vi "Write appended array.vi"(8 "error in (no error)":errorcluster, 10 "appended array":cluster{"AI Channel Data":T1[]}[](array[cluster]), 11 "DAQ Data in":refnum<class "DAQ Data.lvclass">) -> (0 "error out":errorcluster, 3 "DAQ Data out":refnum<class "DAQ Data.lvclass">)   [LabVIEW 2022 SP3, in "DAQ Data.lvclass"]
uses:
  DAQ Data.lvclass
  AIDAQ Data.ctl
  DAQ Data.lvclass/DAQ Data.ctl
  AI Daq Data.lvlib
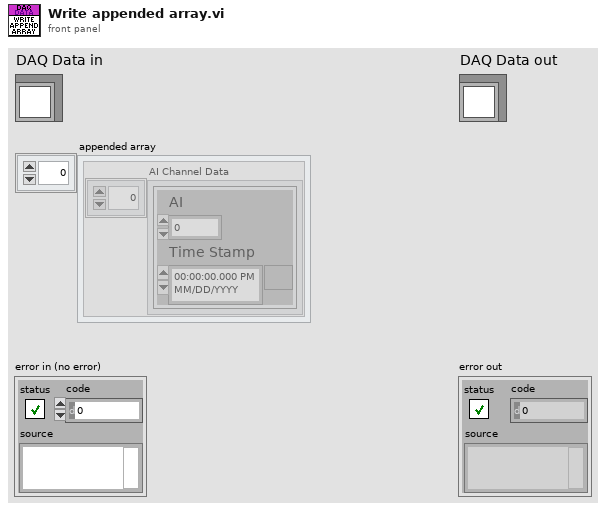
[diagram p1: front panel]
types:
  T1 = typedef "AI Daq Data.lvlib/AIDAQ Data.ctl" = cluster{"AI":dbl, "Time Stamp":timestamp}
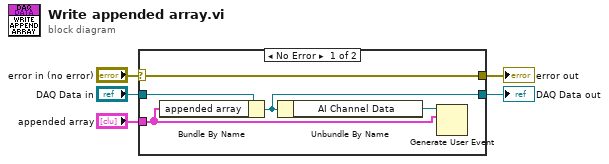
[diagram p0: block diagram]
diagram:
  n1 = case shown="No Error" "error in (no error)" {
    selector: "error in (no error)" -> [w10 w11]
    tunnel: [w10 w11] -> w4
    tunnel: [w8 w12] -> w2
    tunnel: "DAQ Data in" -> [w9 w12]
    tunnel: "appended array" -> [w6 _]
    frame No Error {
      n2 = Bundle By Name(cluster=w9, "appended array"=w6) -> (w8:refnum<class "DAQ Data.lvclass">)
      n3 = Unbundle By Name(w8) -> ("AI Channel Data"=w7:refnum<user-event>)
      n4 = Generate User Event(user event=w7, event data cluster=w6) -> ()  [unwired: 2 in, 2 out]
    }
    frame Error {
    }
  }
  "error out" <- w4
  "DAQ Data out" <- w2
